vi "Write.vi"(8 "error in (no error)":errorcluster, 9 "Variant":variant, 10 "String":string, 11 "VISA in":refnum<class "VISA.lvclass">) -> (0 "error out":errorcluster, 3 "VISA out":refnum<class "VISA.lvclass">)   [LabVIEW 2013, in "Protocol Classes.lvlib" / "VISA.lvclass"]
uses:
  VISA.lvclass
  VISA.lvclass/VISA.ctl
  Read Ref.vi
  Read Append Write Termination Character.vi
  Read Termination Character.vi
  Write Ref.vi
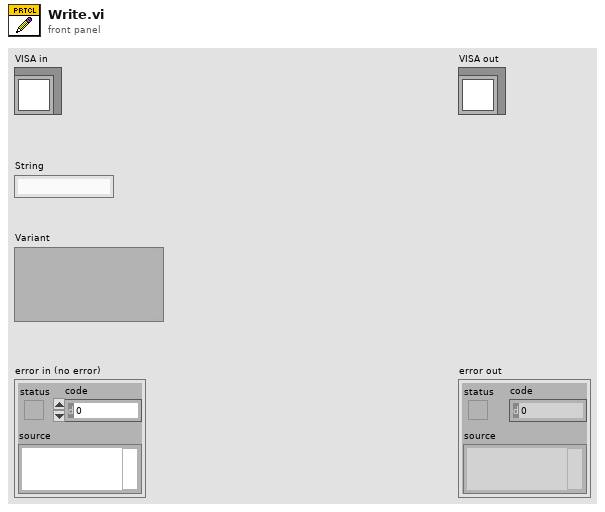
[diagram p1: front panel]
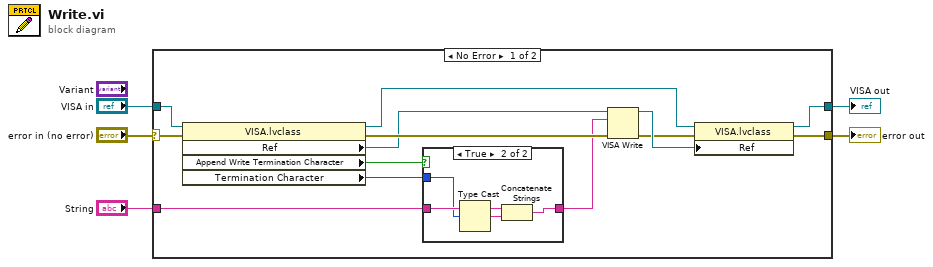
[diagram p0: block diagram]
diagram:
  n1 = case shown="No Error" "error in (no error)" {
    selector: "error in (no error)" -> [w10 w25]
    tunnel: "VISA in" -> [w18 w24]
    tunnel: "String" -> [w8 _]
    tunnel: [w13 w25] -> w2
    tunnel: [w11 w24] -> w1
    frame No Error {
      n2 = property class="VISA.lvclass"(reference=w18, error in=w10) -> (reference out=w12:refnum<class "VISA.lvclass">, error out=w17:errorcluster, "Ref"=w16:refnum<visa-resource-name>, "Append Write Termination Character"=w9:bool, "Termination Character"=w6:u8)
      n3 = case shown="True" w9 {
        tunnel: w8 -> [w19 w23]
        tunnel: [w19 w22] -> w7
        tunnel: w6 -> [_ w21]
        frame False {
        }
        frame True {
          n4 = Type Cast(x=w21) -> (*(type *) &x=w20:string)  [unwired: 1 in]
          n5 = Concatenate Strings(w23, w20) -> (w22:string)
        }
      }
      n6 = VISA Write(VISA resource name=w16, write buffer=w7, error in (no error)=w17) -> (VISA resource name out=w15:refnum<visa-resource-name>, error out=w14:errorcluster)  [unwired: 1 out]
      n7 = property class="VISA.lvclass"(reference=w12, error in=w14, "Ref"=w15) -> (reference out=w11:refnum<class "VISA.lvclass">, error out=w13:errorcluster)
    }
    frame Error {
    }
  }
  "error out" <- w2
  "VISA out" <- w1
